vi "FG MC Loop State (Debug).vi"(1 "FG Action (Read)":T1, 2 "Motor Instruction in":T2={"Motor State"=enum."Stop", "Motor Command"={"Speed"=0, "Turn"=0}}) -> (0 "Motor Instruction out":T2={"Motor State"=enum."Stop", "Motor Command"={"Speed"=0, "Turn"=0}})   [LabVIEW 2009]
uses:
  TypeDefs/Queue TypeDefs/Motor Instruction.ctl
  TypeDefs/Queue TypeDefs/Motor State.ctl
  Remote Control/Motor Command.ctl
  Actions for FG's.ctl
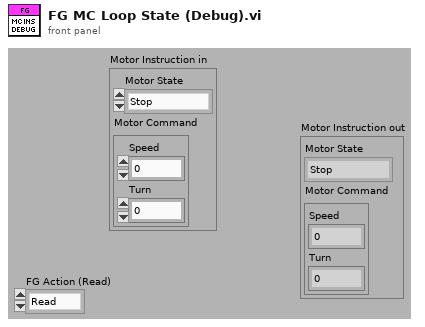
[diagram p1: front panel]
types:
  T1 = typedef "Actions for FG's.ctl" = enum16{"Read", "Write"}
  T2 = typedef "Motor Instruction.ctl" = cluster{"Motor State":T3, "Motor Command":T4}
  T3 = typedef "Motor State.ctl" = enum16{"Wait", "Initialize", "Check FET", "Run", "Stop"}
  T4 = typedef "Motor Command.ctl" = cluster{"Speed":i16, "Turn":i16}
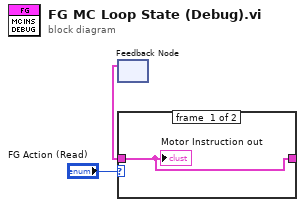
[diagram p0: block diagram]
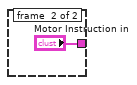
[diagram p2: hidden frame]
diagram:
  n1 = feedback #1() -> (w3:T2)  [unwired: 1 in]
  n2 = case shown="\"Write\"" "FG Action (Read)" {
    tunnel: [w4 "Motor Instruction in"] -> w2
    tunnel: w3 -> [w4 _]
    frame #0 {
      "Motor Instruction out" <- w4
    }
    frame #1 {
    }
  }
